vi "EXCOM-CMD.vi"(0 "VRN IN":refnum<visa-resource-name>="-1", 1 "Bool Refnum":refnum<vi>, 2 "Commande #":i32=-1, 7 "Args":dbl[](array[numeric]) format="%.2f", 11 "Error IN":errorcluster) -> (4 "VRN OUT":refnum<visa-resource-name>="-1", 8 "OK Done":bool, 15 "Error OUT":errorcluster)   [LabVIEW 2019]
uses:
  SerialCommError.vi
panel:
  out "Cmd String":string
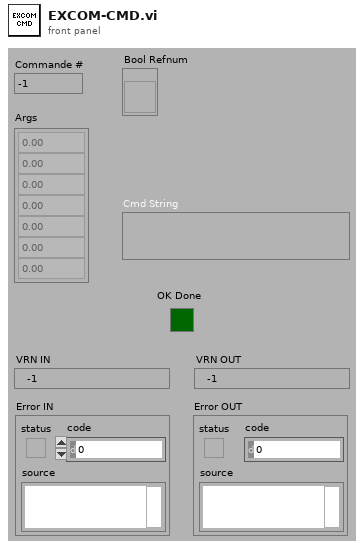
[diagram p1: front panel]
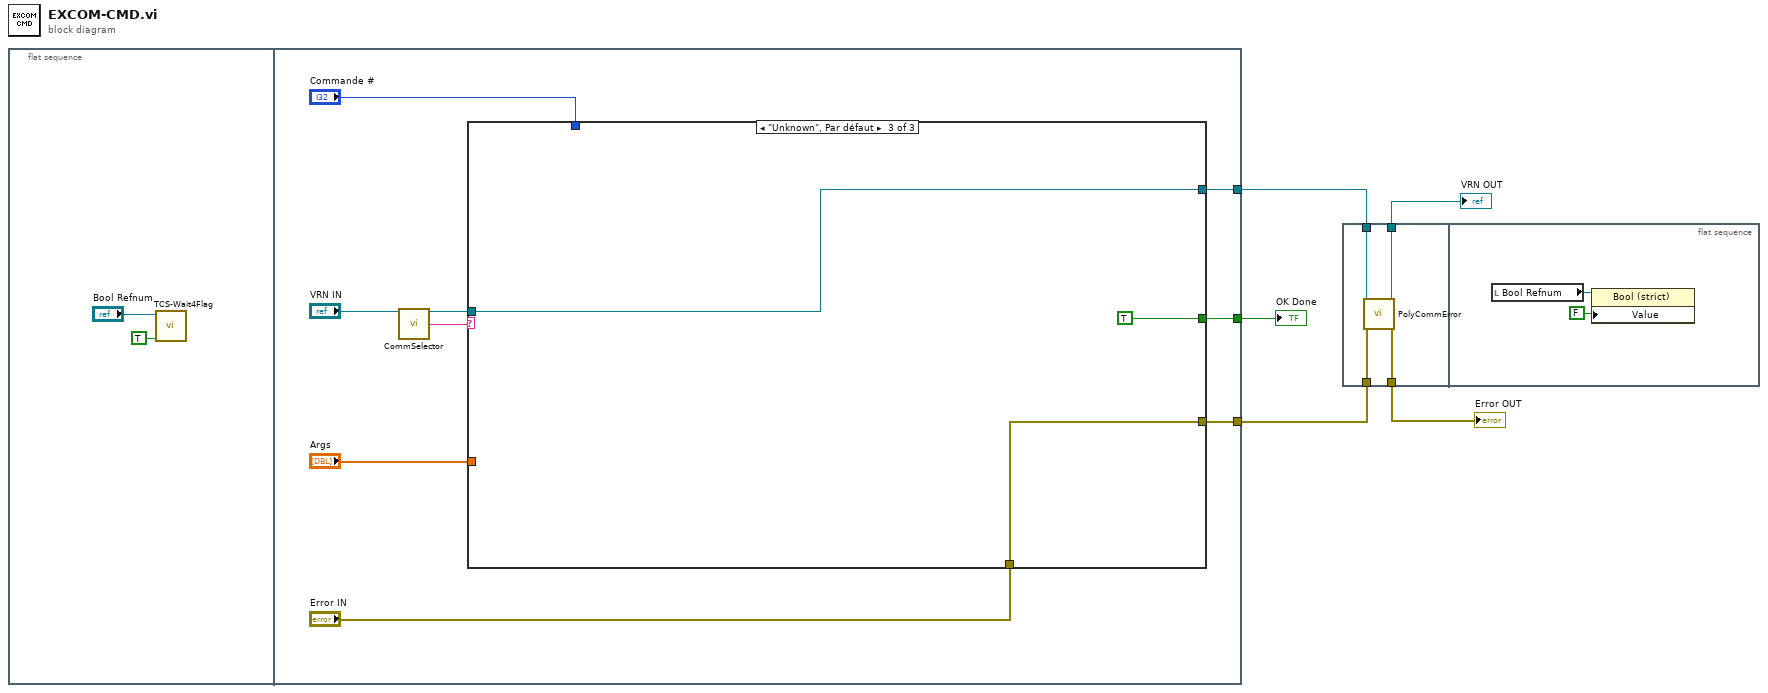
[diagram p0: block diagram]
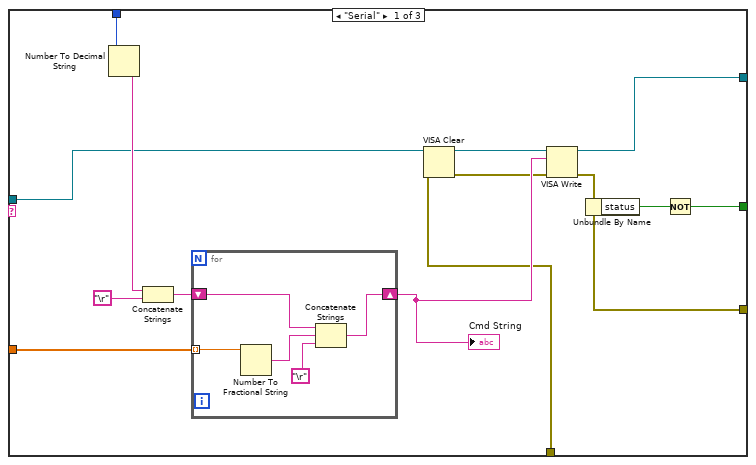
[diagram p2: hidden frame]
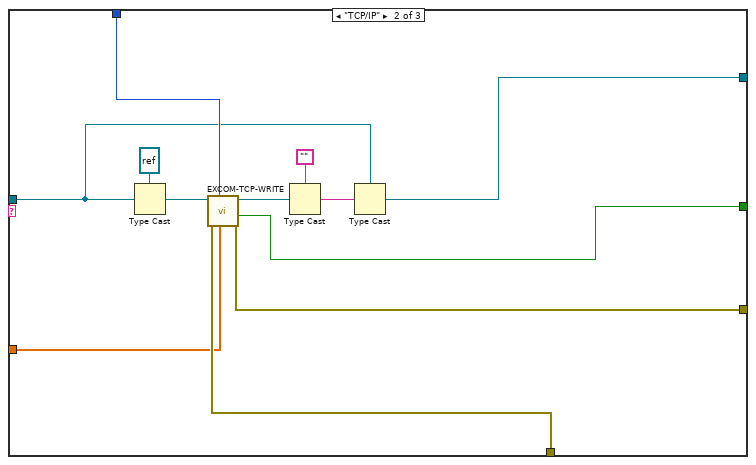
[diagram p3: hidden frame]
diagram:
  n1 = flat-sequence {
    tunnel: [w15] -> w5
    tunnel: [w14] -> w4
    tunnel: [w8] -> w1
    frame #0 {
      n2 = call "TCS-Wait4Flag.vi"("Raise Flag ?"=TRUE, "Ctl Refnum IN"="Bool Refnum") -> ()  [unwired: 8 in, 2 out]
    }
    frame #1 {
      n3 = call "CommSelector.vi"("VISA resource name"="VRN IN") -> ("VISA resource name"=w11:refnum<visa-resource-name>, "CommType"=w12:string)  [unwired: 13 in]
      n4 = case shown="\"Unknown\", Par défaut" w12 {
        tunnel: [w17 w36 TRUE ("status")] -> w8
        tunnel: [w29 w37 w49] -> w14
        tunnel: "Error IN" -> [w24 w45 w49]
        tunnel: [w25 w40 w48] -> w15
        tunnel: w11 -> [w21 w39 w48]
        tunnel: "Commande #" -> [w20 w43 _]
        tunnel: "Args" -> [w19 w44 _]
        frame "Serial" {
          n5 = Number To Decimal String(number=w20) -> (decimal integer string=w27:string)  [unwired: 1 in]
          n6 = Concatenate Strings(w27, "\r") -> (w28:string)
          n7 = for {
            shift-right: [w33] -> w30
            shift-left: w28 -> [w35]
            tunnel: w19 -> [w32] mode=indexing
            n8 = Number To Fractional String(number=w32) -> (F-format string=w31:string)  [unwired: 3 in]
            n9 = Concatenate Strings(w35, w31, "\r") -> (w33:string)
          }
          "Cmd String" <- w30
          n10 = VISA Clear(VISA resource name=w21, error in (no error)=w24) -> (VISA resource name out=w23:refnum<visa-resource-name>, error out=w22:errorcluster)
          n11 = VISA Write(VISA resource name=w23, write buffer=w30, error in (no error)=w22) -> (VISA resource name out=w25:refnum<visa-resource-name>, error out=w29:errorcluster)  [unwired: 1 out]
          n12 = Unbundle By Name(w29) -> ("status"=w18:bool)
          n13 = Not(x=w18) -> (.not. x?=w17:bool)
        }
        frame "TCP/IP" {
          n14 = Type Cast(type=refnum<k5> refnum ("connection ID"), x=w39) -> (*(type *) &x=w46:refnum<k5>)
          n15 = call "EXCOM-TCP-WRITE.vi"("Args"=w44, "Commande #"=w43, "Error IN"=w45, "connection ID"=w46) -> ("Error OUT"=w37:errorcluster, "OK Done"=w36:bool, "connection ID out"=w42:refnum<k5>)  [unwired: 3 in, 1 out]
          n16 = Type Cast(type="", x=w42) -> (*(type *) &x=w41:string)
          n17 = Type Cast(type=w39, x=w41) -> (*(type *) &x=w40:refnum<visa-resource-name>)
        }
        frame "Unknown", Default {
        }
      }
    }
  }
  n18 = flat-sequence {
    tunnel: w5 -> [w54]
    tunnel: w4 -> [w53]
    tunnel: [w52] -> w3
    tunnel: [w51] -> w2
    frame #0 {
      n19 = call-poly "PolyCommError.vi"("VISA IN"=w54, "error IN"=w53) -> ("VISA OUT"=w52:refnum<visa-resource-name>, "error OUT"=w51:errorcluster)  [unwired: 11 in, 1 out]
    }
    frame #1 {
      n20 = local read "Bool Refnum"() -> (w56:refnum<vi>)
      n21 = property on="Property Node" class="Bool (strict)"(reference=w56, "Value"=FALSE ("Raise Flag ?")) -> ()  [unwired: 1 in, 2 out]
    }
  }
  "OK Done" <- w1
  "VRN OUT" <- w3
  "Error OUT" <- w2
